vi "Automatic Teller Machine (ATM).vi"() -> ()   [LabVIEW 2020]
doc: "This VI simulates the behavior of an Automated Teller Machine (ATM)."
uses:
  Controls/Machine States.ctl
  Controls/Controls-Indicators References.ctl
  Controls/ATM Message Types.ctl
  Controls/Previous State.ctl
panel:
  in  "Enter":bool
  in  "User Input":string
  in  "Right Buttons":T1
  out "Right Menu":T2
  in  "Left Buttons":T1
  out "Left Menu":T2
  in  "Card Simulator":bool
  out "ATM Messages":string
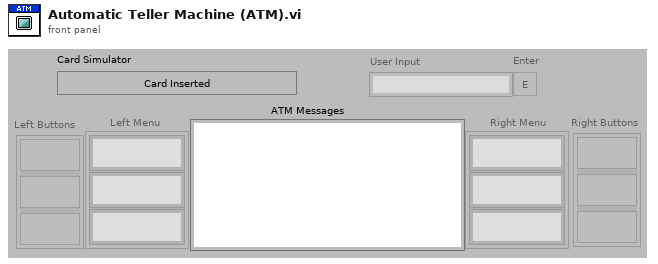
[diagram p1: front panel]
types:
  T1 = cluster{"Func Button":bool, "Func Button 2":bool, "Func Button 3":bool}
  T2 = cluster{"RFS String":string, "RFS String 2":string, "RFS String 3":string}
  T3 = typedef "Controls-Indicators References.ctl" = cluster{"Enter":refnum<vi>, "User Input":refnum<vi>, "Right Buttons":refnum<vi>, "Right Menu":refnum<vi>, "Left Buttons":refnum<vi>, "Left Menu":refnum<vi>, "Card Simulator":refnum<vi>, "ATM Messages":refnum<vi>}
  T4 = typedef "Machine States.ctl" = enum16{"Initialize", "Account Verification", "Deposit", "Withdraw", "None", "Fast Cash", "Balance Inquiry", "Wait User Action", "Return Card"}
  T5 = typedef "Previous State.ctl" = enum16{"Initialize", "Wait User Action", "Account Verification", "Wait Withdraw", "Wait Deposit"}
  T6 = typedef "ATM Message Types.ctl" = enum16{"Welcome", "Main Menu", "Account Verification Failed", "Session Terminate Message", "Deposit ", "Deposit Completed", "Withdrawal", "Withdrawal Complete", "Withdrawal Failed", "Balance Inquiry"}
  T7 = cluster{"Balance":dbl, "Name":string, "Password":string}
  T8 = enum8{"Enabled", "Disabled", "Disabled and Grayed Out"}
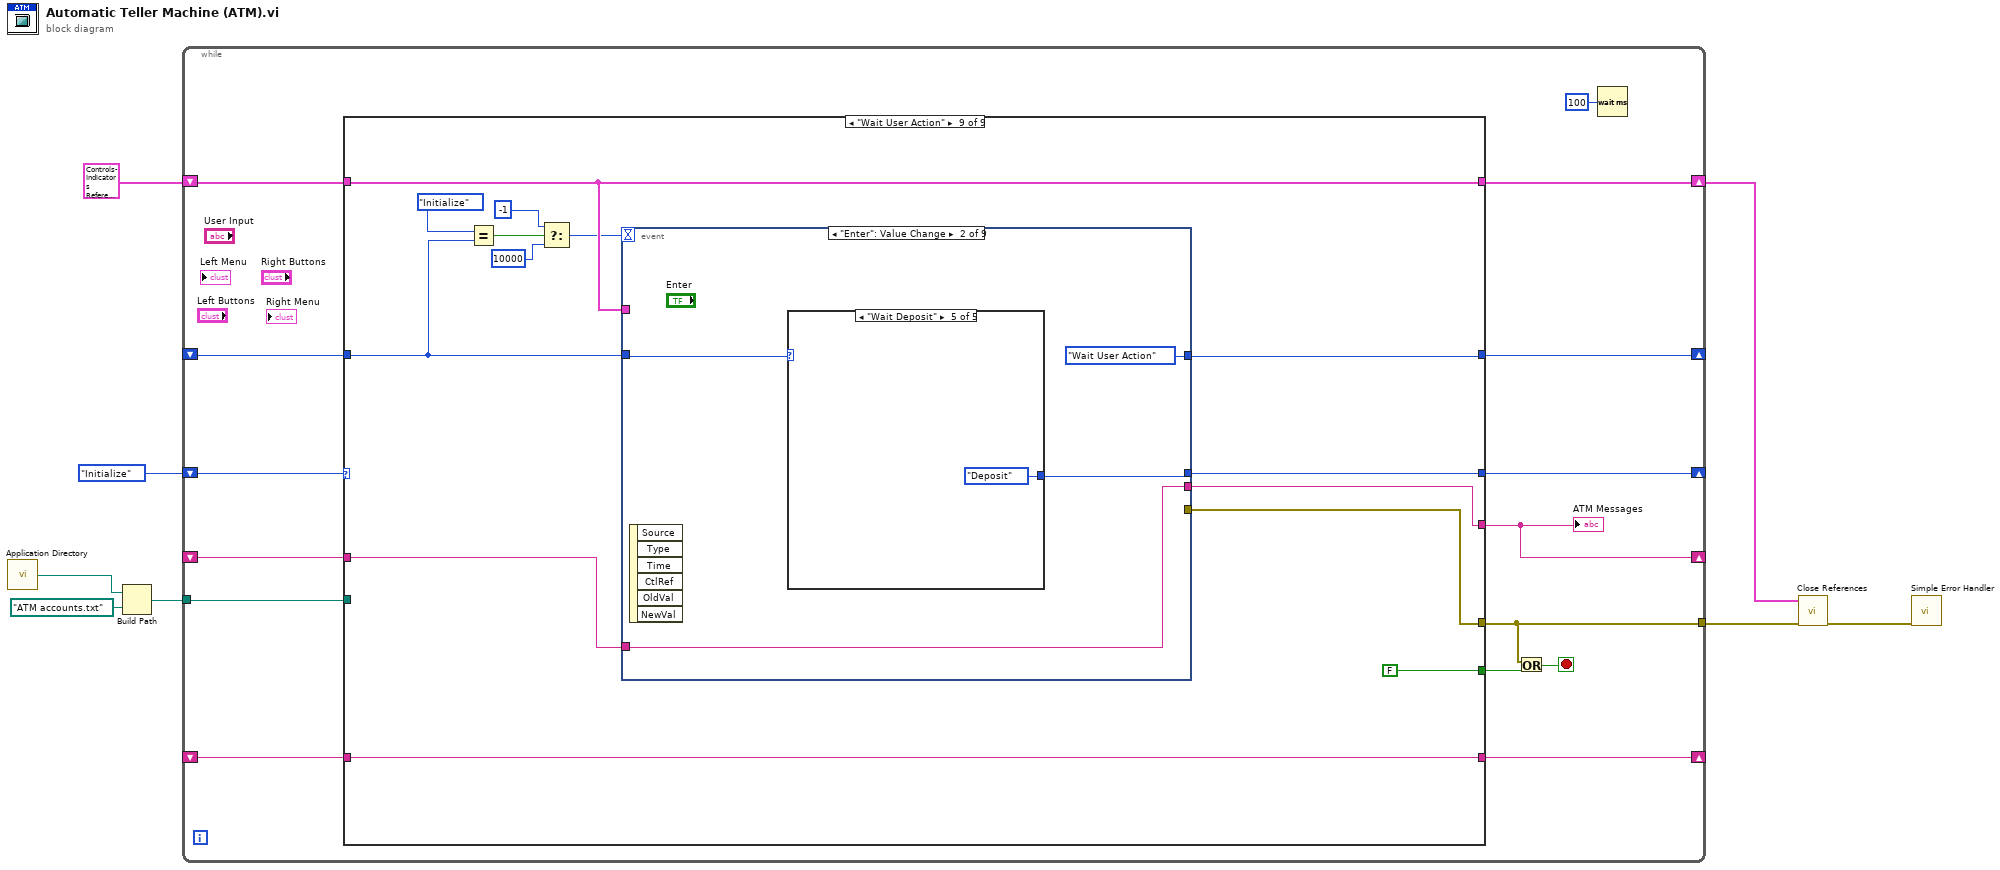
[diagram p0: block diagram]
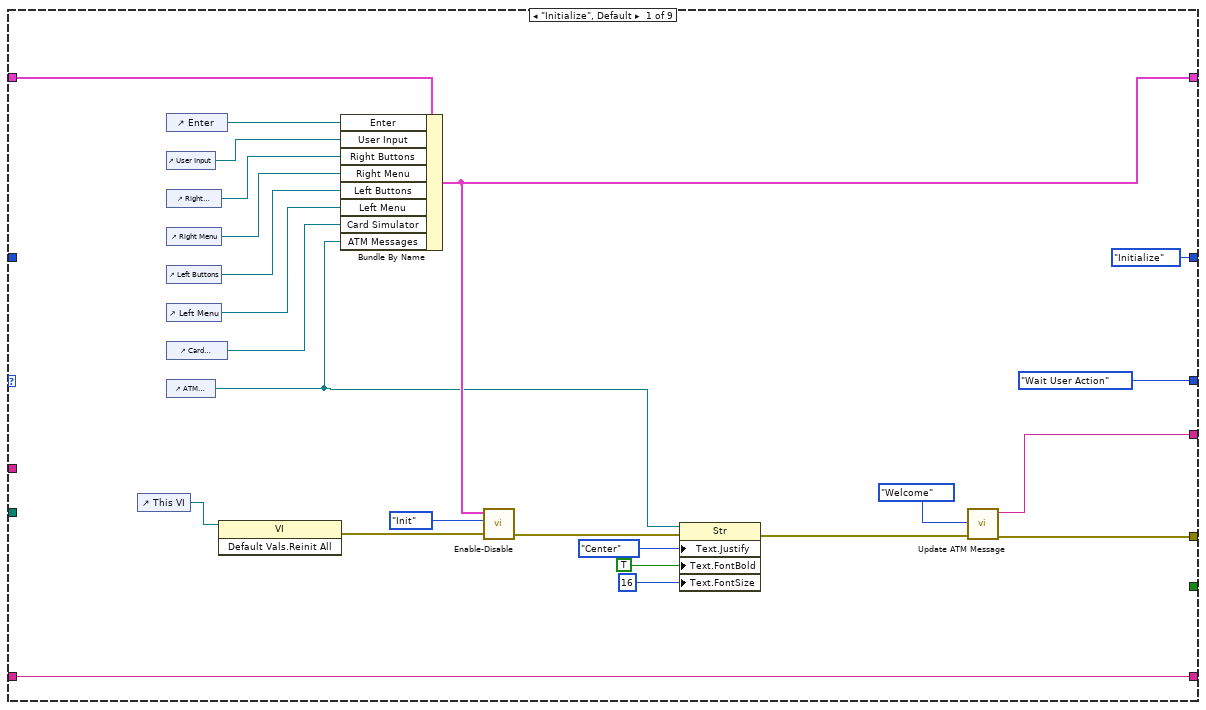
[diagram p2: hidden frame]
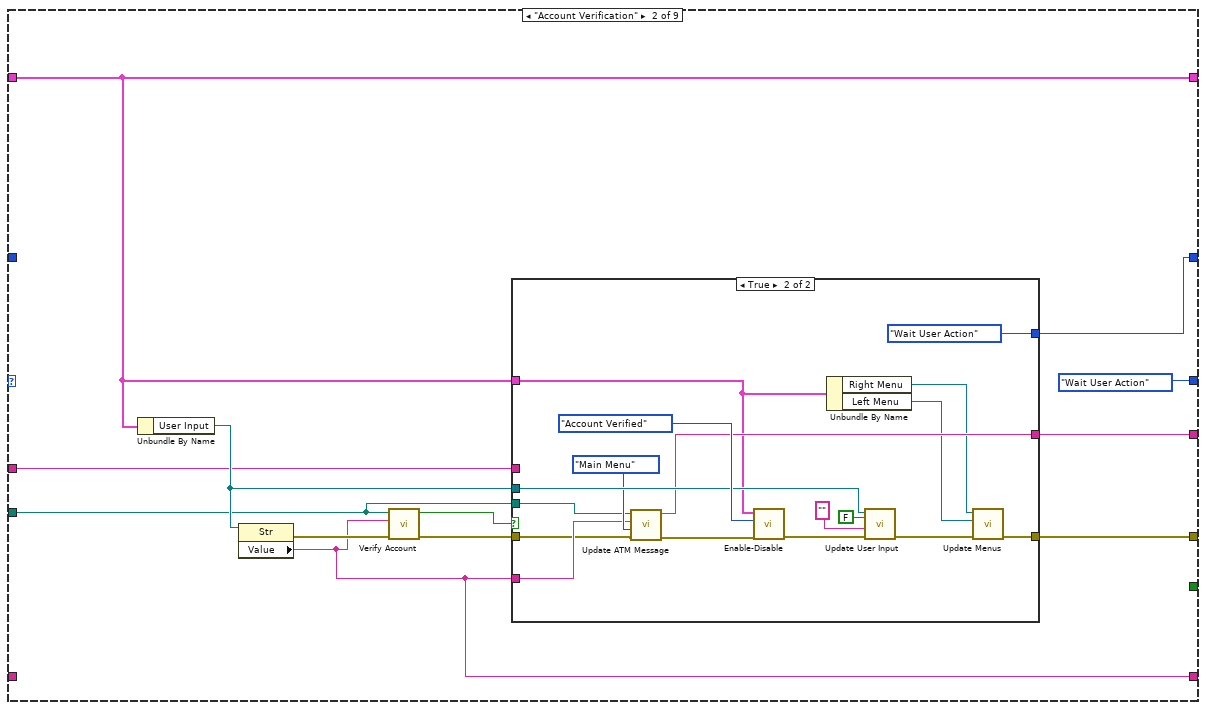
[diagram p3: hidden frame]
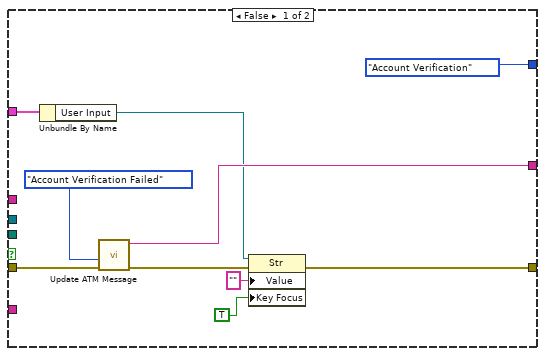
[diagram p4: hidden frame]
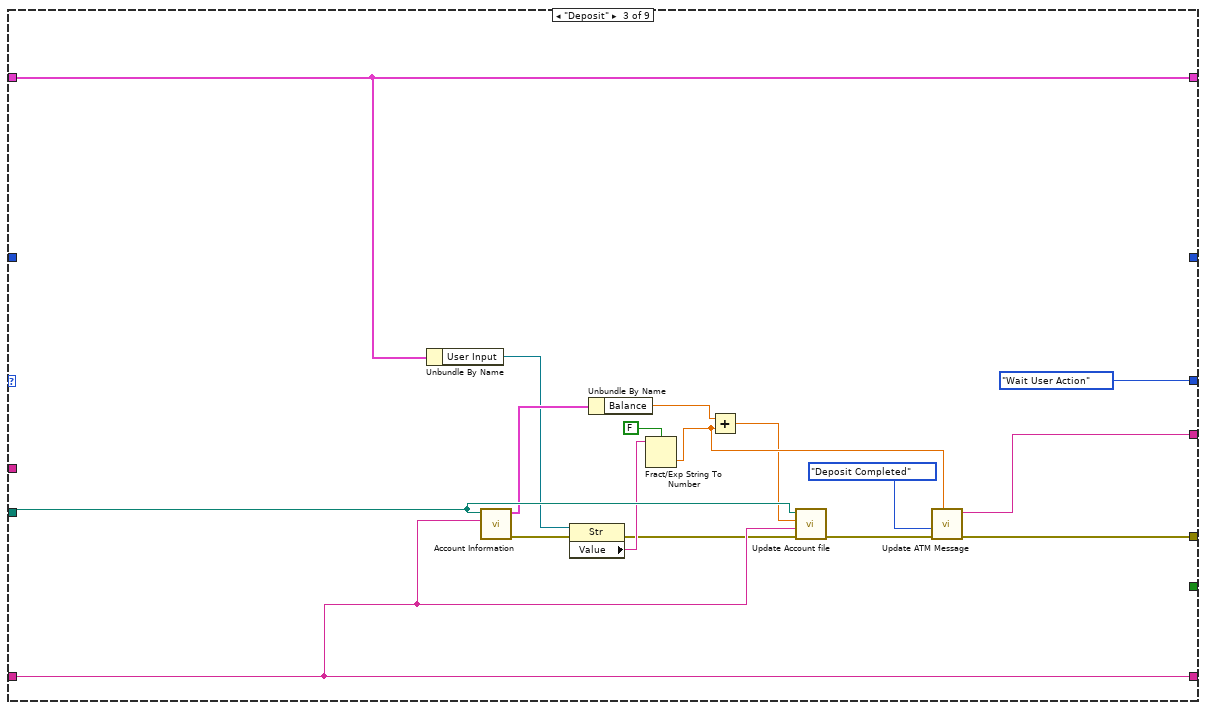
[diagram p5: hidden frame]
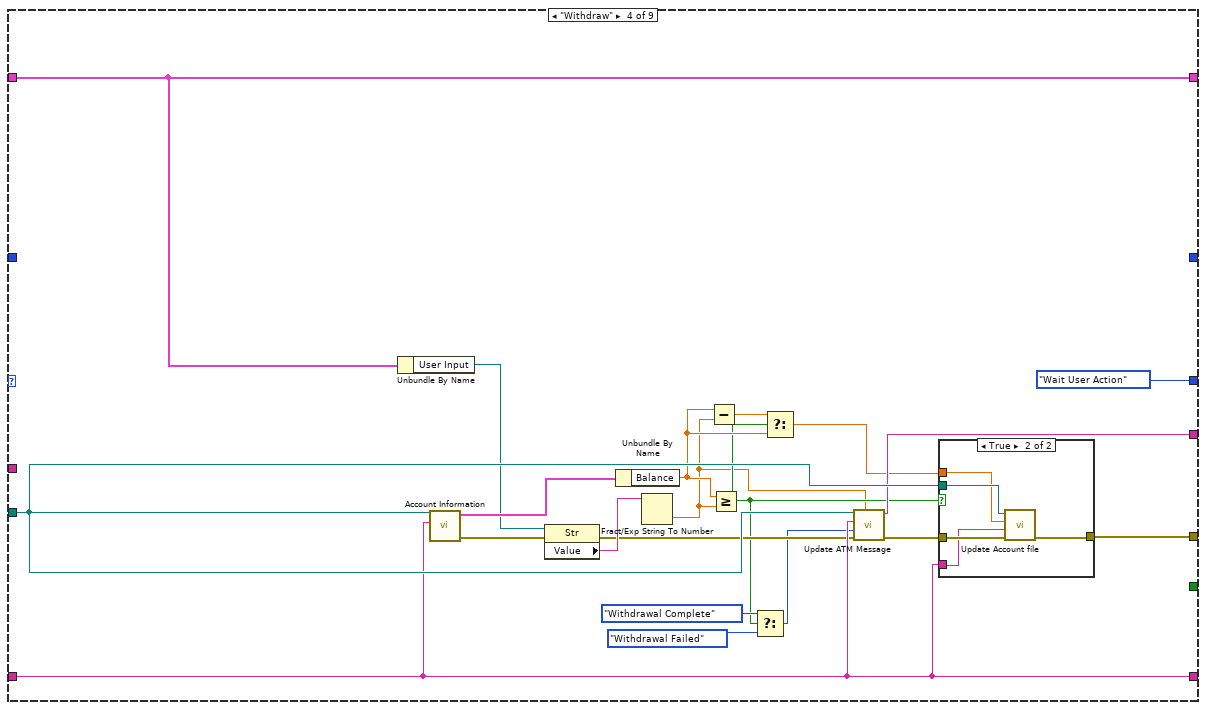
[diagram p6: hidden frame]
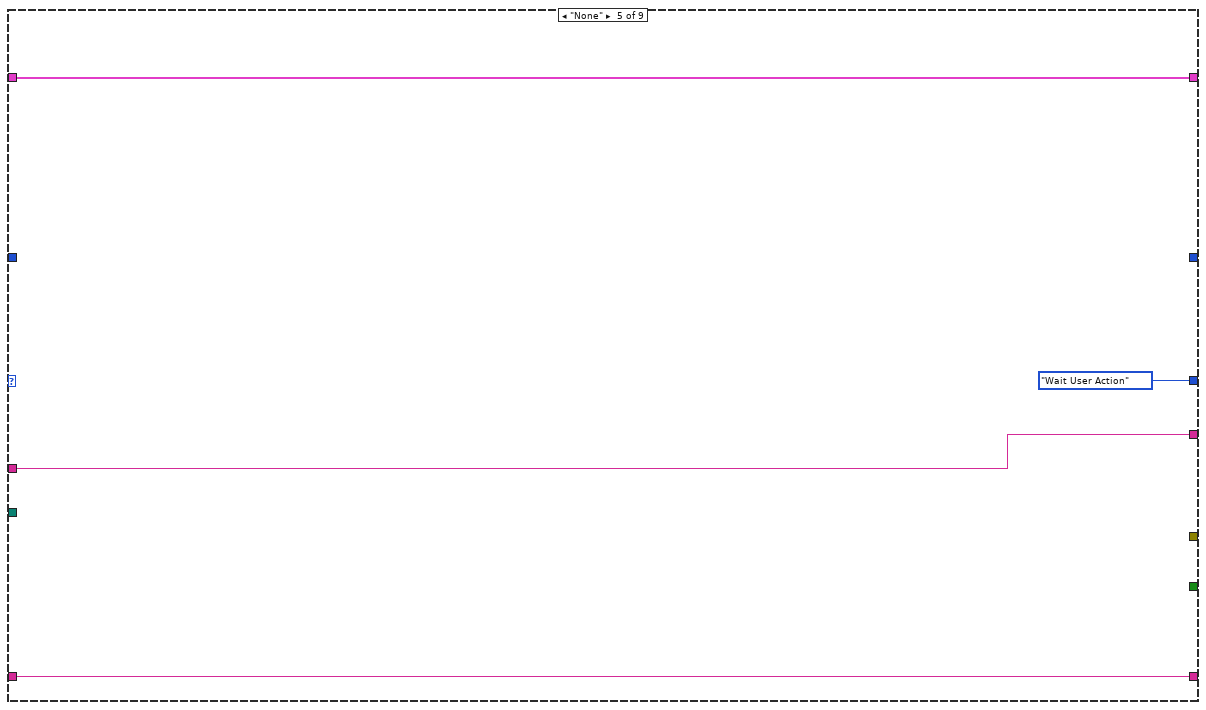
[diagram p8: hidden frame]
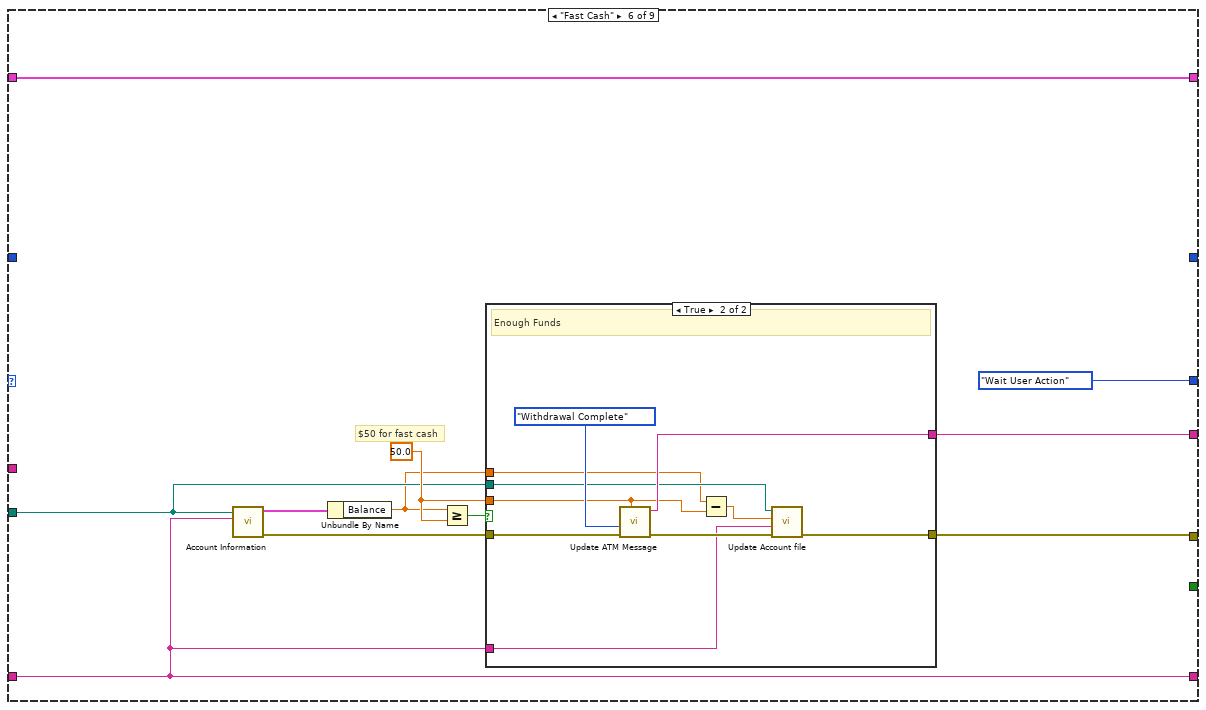
[diagram p9: hidden frame]
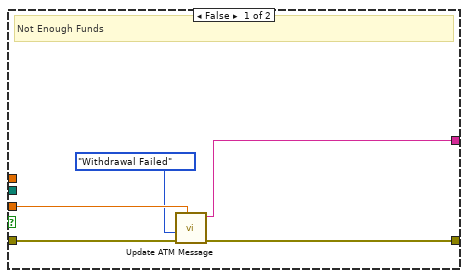
[diagram p10: hidden frame]
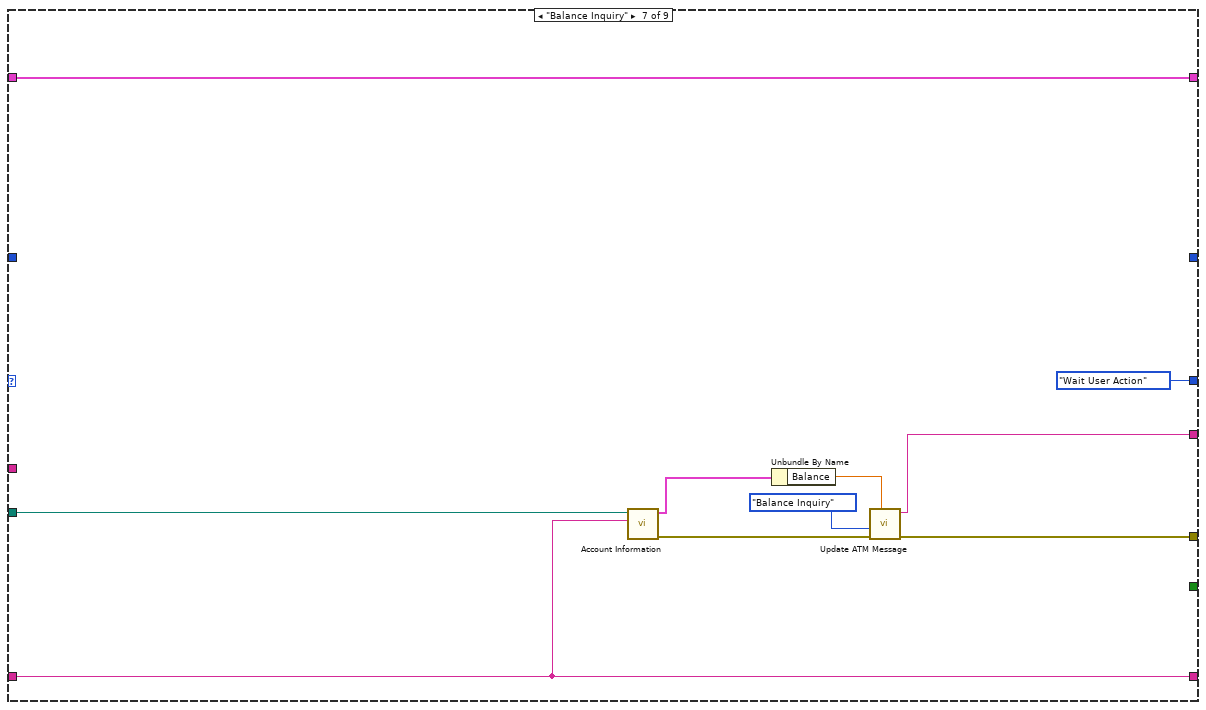
[diagram p11: hidden frame]
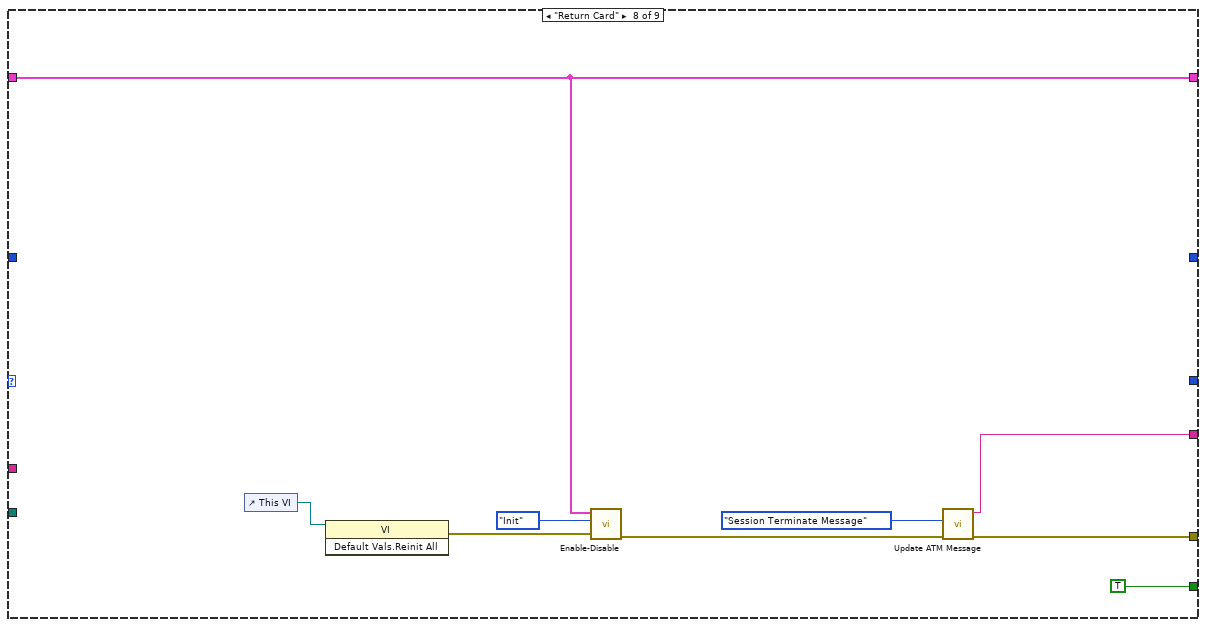
[diagram p12: hidden frame]
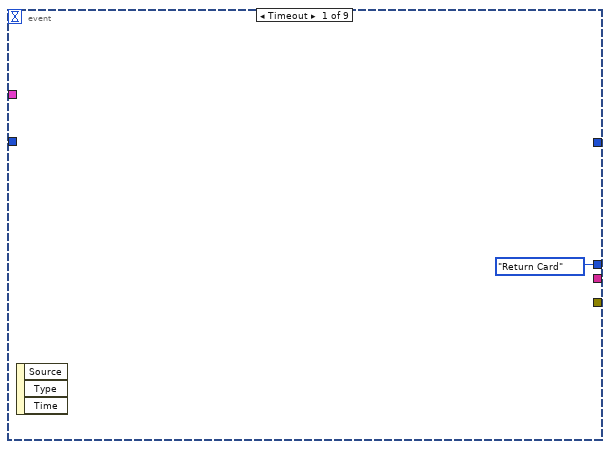
[diagram p13: hidden frame]
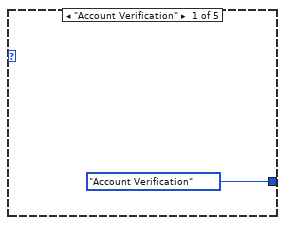
[diagram p14: hidden frame]
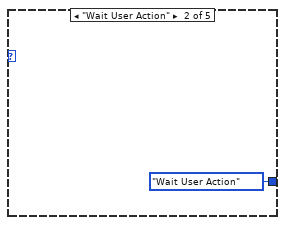
[diagram p15: hidden frame]
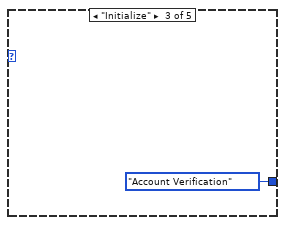
[diagram p16: hidden frame]
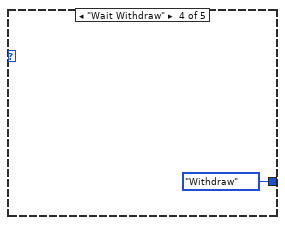
[diagram p17: hidden frame]
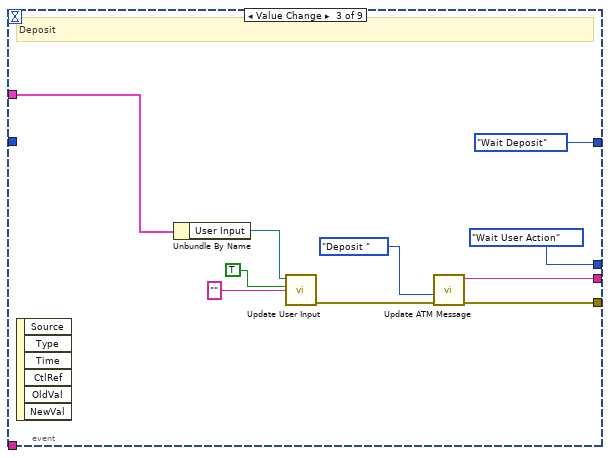
[diagram p18: hidden frame]
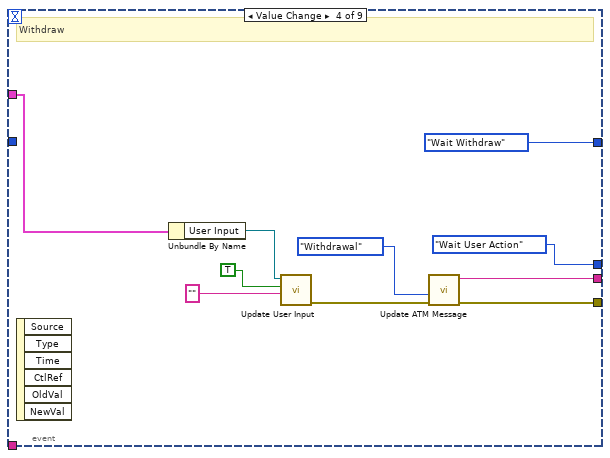
[diagram p19: hidden frame]
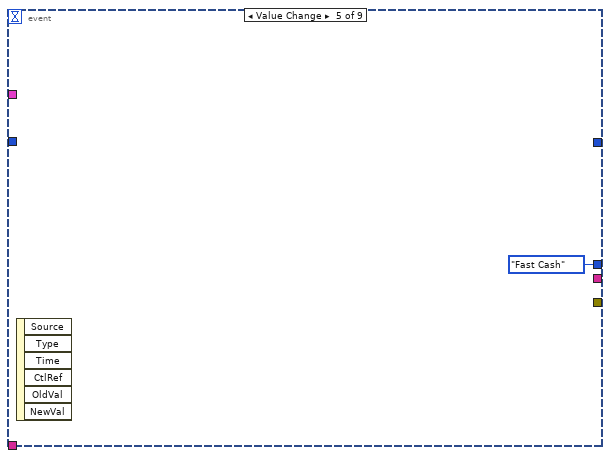
[diagram p20: hidden frame]
diagram:
  n1 = call <vilib>:"Application Directory.vi"() -> ("Application Directory"=w4:path)
  n2 = Build Path(base path=w4, name or relative path=path "ATM accounts.txt") -> (appended path=w5:path)
  n3 = while {
    shift-right: [w19] -> _
    shift-left: Machine_States."Initialize" ("Enum") -> [w23]
    shift-right: [w18] -> _
    shift-left: _ -> [w17]
    shift-right: [w20] -> w3
    shift-left: T3 {"Enter"=refnum, "User Input"=refnum, "Right Buttons"=refnum, "Right Menu"=refnum, "Left Buttons"=refnum, "Left Menu"=refnum, "Card Simulator"=refnum, "ATM Messages"=refnum} ("input cluster") -> [w21]
    tunnel: w5 -> [w16]
    shift-right: [w14] -> _
    shift-left: _ -> [w13]
    shift-right: [w10] -> _
    shift-left: _ -> [w11]
    tunnel: [w9] -> w2
    stop <- w22 stop-if-true
    n4 = case shown="\"Wait User Action\"" w23 {
      tunnel: [w45 w56 w102 w120 _ w135 w168 w177 w188] -> w9
      tunnel: w21 -> [w47 w51 w99 w121 w133 w144 w169 w170 w190]
      tunnel: [w44 w51 w99 w121 w133 w144 w169 w170 w190] -> w20
      tunnel: [w46 w53 w101 w119 w131 w139 w160 w176 w180] -> w18
      tunnel: [Machine_States."Wait User Action" ("Enum") Machine_States."Wait User Action" ("Enum") Machine_States."Wait User Action" ("Enum") Machine_States."Wait User Action" ("Enum") Machine_States."Wait User Action" ("Enum") Machine_States."Wait User Action" ("Enum") Machine_States."Wait User Action" ("Enum") _ w192] -> w19
      tunnel: w17 -> [_ w52 _ _ w131 _ _ _ w179]
      tunnel: w16 -> [_ w54 w103 w123 _ w138 w165 _ _]
      tunnel: [_ _ _ _ _ _ _ TRUE ("x .or. y?") FALSE ("x .or. y?")] -> w15
      tunnel: [w25 w50 w98 w122 w132 w137 w166 _ w189] -> w14
      tunnel: w13 -> [w25 _ w98 w122 w132 w137 w166 _ w189]
      tunnel: w11 -> [_ _ _ _ _ _ _ _ w187]
      tunnel: [Previous_State."Initialize" w49 _ _ _ _ _ _ w181] -> w10
      frame "Initialize", Default {
        n5 = control-ref of="This VI"() -> (w41:refnum<vi>)
        n6 = control-ref of="Enter"() -> (w32:refnum<vi>)
        n7 = control-ref of="User Input"() -> (w31:refnum<vi>)
        n8 = control-ref of="Right Buttons"() -> (w30:refnum<vi>)
        n9 = control-ref of="Right Menu"() -> (w29:refnum<vi>)
        n10 = control-ref of="Left Buttons"() -> (w28:refnum<vi>)
        n11 = control-ref of="Left Menu"() -> (w27:refnum<vi>)
        n12 = control-ref of="Card Simulator"() -> (w26:refnum<vi>)
        n13 = control-ref of="ATM Messages"() -> (w43:refnum<vi>)
        n14 = invoke class="VI" method="Default Vals.Reinit All"(reference=w41) -> (error out=w40:errorcluster)  [unwired: 2 in, 2 out]
        n15 = Bundle By Name(cluster=w47, "Enter"=w32, "User Input"=w31, "Right Buttons"=w30, "Right Menu"=w29, "Left Buttons"=w28, "Left Menu"=w27, "Card Simulator"=w26, "ATM Messages"=w43) -> (w44:T3)
        n16 = call "Enable-Disable.vi"("error in (no error)"=w40, "State"=enum16{"Init", "Account Verified"}."Init", "Control/Indicator References"=w44) -> ("error out"=w38:errorcluster)  [unwired: 8 in]
        n17 = property class="Str"(reference=w43, error in=w38, "Text.Justify"=enum16{"Left", "Center", "Right"}."Center" ("Text.Justification"), "Text.FontBold"=TRUE ("Text.Font:Bold"), "Text.FontSize"=u32 16 ("Text.Font:Size")) -> (error out=w33:errorcluster)  [unwired: 1 out]
        n18 = call "Update ATM Message.vi"("error in (no error)"=w33, "ATM Message Type"=ATM_Message_Types."Welcome") -> ("error out"=w45:errorcluster, "ATM Messages"=w46:string)  [unwired: 8 in]
      }
      frame "Account Verification" {
        n19 = Unbundle By Name(w51) -> ("User Input"=w55:refnum<vi>)
        n20 = property class="Str"(reference=w55) -> (error out=w59:errorcluster, "Value"=w50:string)  [unwired: 1 in, 1 out]
        n21 = call "Verify Account.vi"("error in (no error)"=w59, "Account"=w50, "Path Account File"=w54) -> ("error out"=w57:errorcluster, "Account exist?"=w58:bool)  [unwired: 7 in]
        n22 = case shown="True" w58 {
          tunnel: w57 -> [w66 w79]
          tunnel: [w61 w74] -> w56
          tunnel: w55 -> [_ w84]
          tunnel: w54 -> [_ w82]
          tunnel: w50 -> [_ w81]
          tunnel: [w67 w80] -> w53
          tunnel: w52 -> [_ _]
          tunnel: w51 -> [w69 w73]
          tunnel: [Previous_State."Account Verification" Previous_State."Wait User Action"] -> w49
          frame False {
            n23 = Unbundle By Name(w69) -> ("User Input"=w64:refnum<vi>)
            n24 = call "Update ATM Message.vi"("error in (no error)"=w66, "ATM Message Type"=ATM_Message_Types."Account Verification Failed") -> ("error out"=w65:errorcluster, "ATM Messages"=w67:string)  [unwired: 8 in]
            n25 = property class="Str"(reference=w64, error in=w65, "Value"="", "Key Focus"=TRUE) -> (error out=w61:errorcluster)  [unwired: 1 out]
          }
          frame True {
            n26 = call "Update ATM Message.vi"("error in (no error)"=w79, "ATM Message Type"=ATM_Message_Types."Main Menu", "Password"=w81, "Path Account File"=w82) -> ("error out"=w78:errorcluster, "ATM Messages"=w80:string)  [unwired: 6 in]
            n27 = call "Enable-Disable.vi"("error in (no error)"=w78, "State"=enum16{"Init", "Account Verified"}."Account Verified", "Control/Indicator References"=w73) -> ("error out"=w85:errorcluster)  [unwired: 8 in]
            n28 = Unbundle By Name(w73) -> ("Right Menu"=w72:refnum<vi>, "Left Menu"=w71:refnum<vi>)
            n29 = call "Update User Input.vi"("error in (no error)"=w85, "Value"="", "Key Focus"=FALSE, "User Input Reference"=w84) -> ("error out"=w75:errorcluster)  [unwired: 7 in]
            n30 = call "Update Menus.vi"("error in (no error)"=w75, "Left Menu"=w71, "Right Menu"=w72) -> ("error out"=w74:errorcluster)  [unwired: 8 in]
          }
        }
      }
      frame "Deposit" {
        n31 = Unbundle By Name(w99) -> ("User Input"=w96:refnum<vi>)
        n32 = call "Account Information.vi"("Password"=w98, "file path (dialog if empty)"=w103) -> ("error out"=w93:errorcluster, "Account Information"=w97:T7)  [unwired: 8 in]
        n33 = property class="Str"(reference=w96, error in=w93) -> (error out=w92:errorcluster, "Value"=w95:string)  [unwired: 1 out]
        n34 = Unbundle By Name(w97) -> ("Balance"=w91:dbl)
        n35 = Fract/Exp String To Number(use system decimal point (T)=FALSE, string=w95) -> (number=w88:dbl)  [unwired: 2 in, 1 out]
        n36 = Add(x=w91, y=w88) -> (x+y=w87:dbl)
        n37 = call "Update Account file.vi"("error in (no error)"=w92, "Account"=w98, "Balance"=w87, "name or relative path"=w103) -> ("error out"=w94:errorcluster)  [unwired: 7 in]
        n38 = call "Update ATM Message.vi"("Balance"=w88, "error in (no error)"=w94, "ATM Message Type"=ATM_Message_Types."Deposit Completed") -> ("error out"=w102:errorcluster, "ATM Messages"=w101:string)  [unwired: 7 in]
      }
      frame "Withdraw" {
        n39 = Unbundle By Name(w121) -> ("User Input"=w116:refnum<vi>)
        n40 = call "Account Information.vi"("Password"=w122, "file path (dialog if empty)"=w123) -> ("error out"=w117:errorcluster, "Account Information"=w118:T7)  [unwired: 8 in]
        n41 = property class="Str"(reference=w116, error in=w117) -> (error out=w114:errorcluster, "Value"=w115:string)  [unwired: 1 out]
        n42 = Unbundle By Name(w118) -> ("Balance"=w109:dbl)
        n43 = Fract/Exp String To Number(string=w115) -> (number=w104:dbl)  [unwired: 3 in, 1 out]
        n44 = Subtract(x=w109, y=w104) -> (x-y=w110:dbl)
        n45 = Greater Or Equal?(x=w109, y=w104) -> (x >= y?=w108:bool)
        n46 = Select(t=ATM_Message_Types."Withdrawal Complete" ("ATM Message Type"), s=w108, f=ATM_Message_Types."Withdrawal Failed" ("ATM Message Type")) -> (s? t:f=w111:T6)
        n47 = Select(t=w110, s=w108, f=w109) -> (s? t:f=w105:dbl)
        n48 = call "Update ATM Message.vi"("Balance"=w104, "error in (no error)"=w114, "ATM Message Type"=w111, "Password"=w122, "Path Account File"=w123) -> ("error out"=w107:errorcluster, "ATM Messages"=w119:string)  [unwired: 5 in]
        n49 = case shown="True" w108 {
          tunnel: w107 -> [w124 w129]
          tunnel: [w124 w128] -> w120
          tunnel: w123 -> [_ w127]
          tunnel: w105 -> [_ w126]
          tunnel: w122 -> [_ w125]
          frame False {
          }
          frame True {
            n50 = call "Update Account file.vi"("error in (no error)"=w129, "Account"=w125, "Balance"=w126, "name or relative path"=w127) -> ("error out"=w128:errorcluster)  [unwired: 7 in]
          }
        }
      }
      frame "None" {
      }
      frame "Fast Cash" {
        w140 = 50.0 ("y")
        # "$50 for fast cash"
        n51 = call "Account Information.vi"("Password"=w137, "file path (dialog if empty)"=w138) -> ("error out"=w142:errorcluster, "Account Information"=w143:T7)  [unwired: 8 in]
        n52 = Unbundle By Name(w143) -> ("Balance"=w136:dbl)
        n53 = Greater Or Equal?(x=w136, y=w140) -> (x >= y?=w141:bool)
        n54 = case shown="True" w141 {
          tunnel: w142 -> [w149 w158]
          tunnel: w140 -> [w148 w150]
          tunnel: [w146 w157] -> w139
          tunnel: [w145 w155] -> w135
          tunnel: w138 -> [_ w154]
          tunnel: w137 -> [_ w153]
          tunnel: w136 -> [_ w151]
          frame False {
            # "Not Enough Funds"
            n55 = call "Update ATM Message.vi"("Balance"=w148, "error in (no error)"=w149, "ATM Message Type"=ATM_Message_Types."Withdrawal Failed") -> ("error out"=w145:errorcluster, "ATM Messages"=w146:string)  [unwired: 7 in]
          }
          frame True {
            # "Enough Funds"
            n56 = call "Update ATM Message.vi"("Balance"=w150, "error in (no error)"=w158, "ATM Message Type"=ATM_Message_Types."Withdrawal Complete") -> ("error out"=w156:errorcluster, "ATM Messages"=w157:string)  [unwired: 7 in]
            n57 = Subtract(x=w151, y=w150) -> (x-y=w152:dbl)
            n58 = call "Update Account file.vi"("error in (no error)"=w156, "Account"=w153, "Balance"=w152, "name or relative path"=w154) -> ("error out"=w155:errorcluster)  [unwired: 7 in]
          }
        }
      }
      frame "Balance Inquiry" {
        n59 = call "Account Information.vi"("Password"=w166, "file path (dialog if empty)"=w165) -> ("error out"=w167:errorcluster, "Account Information"=w164:T7)  [unwired: 8 in]
        n60 = Unbundle By Name(w164) -> ("Balance"=w163:dbl)
        n61 = call "Update ATM Message.vi"("Balance"=w163, "error in (no error)"=w167, "ATM Message Type"=ATM_Message_Types."Balance Inquiry") -> ("error out"=w168:errorcluster, "ATM Messages"=w160:string)  [unwired: 7 in]
      }
      frame "Return Card" {
        n62 = control-ref of="This VI"() -> (w174:refnum<vi>)
        n63 = invoke class="VI" method="Default Vals.Reinit All"(reference=w174) -> (error out=w173:errorcluster)  [unwired: 2 in, 2 out]
        n64 = call "Enable-Disable.vi"("error in (no error)"=w173, "State"=enum16{"Init", "Account Verified"}."Init", "Control/Indicator References"=w170) -> ("error out"=w171:errorcluster)  [unwired: 8 in]
        n65 = call "Update ATM Message.vi"("error in (no error)"=w171, "ATM Message Type"=ATM_Message_Types."Session Terminate Message") -> ("error out"=w177:errorcluster, "ATM Messages"=w176:string)  [unwired: 8 in]
      }
      frame "Wait User Action" {
        n66 = Equal?(x=Previous_State."Initialize", y=w187) -> (x = y?=w185:bool)
        n67 = Select(t=-1, s=w185, f=10000) -> (s? t:f=w182:i32)
        n68 = event shown="[1] \"Enter\": Value Change" {
          selector: _ -> [_ _ _ _ _ _ _ _ _]
          dyn-events: _ -> [_ _ _ _ _ _ _ _ _]
          timeout: w182 -> [_ _ _ _ _ _ _ _ _]
          tunnel: w190 -> [_ _ w206 w214 _ _ _ _ w231]
          tunnel: [Machine_States."Return Card" ("Enum") w196 Machine_States."Wait User Action" ("Enum") Machine_States."Wait User Action" ("Enum") Machine_States."Fast Cash" ("Enum") Machine_States."None" ("Enum") Machine_States."Balance Inquiry" ("Enum") Machine_States."Return Card" ("Enum") Machine_States."Wait User Action" ("Enum")] -> w192
          tunnel: w187 -> [_ w197 _ _ _ _ _ _ _]
          tunnel: [_ _ w207 w218 _ _ _ _ w232] -> w188
          tunnel: [_ Previous_State."Wait User Action" Previous_State."Wait Deposit" Previous_State."Wait Withdraw" _ _ _ _ Previous_State."Account Verification"] -> w181
          tunnel: [_ w195 w205 w217 _ w224 _ _ w228] -> w180
          tunnel: w179 -> [_ w195 _ _ _ w224 _ _ w228]
          event Timeout {
            n69 = event-data() -> ()  [unwired: 1 in, 3 out]
          }
          event "Enter": Value Change {
            n70 = event-data() -> ()  [unwired: 1 in, 6 out]
            n71 = case shown="\"Wait Deposit\"" w197 {
              tunnel: [Machine_States."Account Verification" ("Enum") Machine_States."Wait User Action" ("Enum") Machine_States."Account Verification" ("Enum") Machine_States."Withdraw" ("Enum") Machine_States."Deposit" ("Enum")] -> w196
              frame "Account Verification" {
              }
              frame "Wait User Action" {
              }
              frame "Initialize" {
              }
              frame "Wait Withdraw" {
              }
              frame "Wait Deposit" {
              }
            }
          }
          event "Right Buttons.Func Button": Value Change {
            # "Deposit"
            n72 = event-data() -> ()  [unwired: 1 in, 6 out]
            n73 = Unbundle By Name(w206) -> ("User Input"=w210:refnum<vi>)
            n74 = call "Update User Input.vi"("Value"="", "Key Focus"=TRUE, "User Input Reference"=w210) -> ("error out"=w211:errorcluster)  [unwired: 8 in]
            n75 = call "Update ATM Message.vi"("error in (no error)"=w211, "ATM Message Type"=ATM_Message_Types."Deposit ") -> ("error out"=w207:errorcluster, "ATM Messages"=w205:string)  [unwired: 8 in]
          }
          event "Right Buttons.Func Button 2": Value Change {
            # "Withdraw"
            n76 = event-data() -> ()  [unwired: 1 in, 6 out]
            n77 = Unbundle By Name(w214) -> ("User Input"=w213:refnum<vi>)
            n78 = call "Update User Input.vi"("Value"="", "Key Focus"=TRUE, "User Input Reference"=w213) -> ("error out"=w221:errorcluster)  [unwired: 8 in]
            n79 = call "Update ATM Message.vi"("error in (no error)"=w221, "ATM Message Type"=ATM_Message_Types."Withdrawal") -> ("error out"=w218:errorcluster, "ATM Messages"=w217:string)  [unwired: 8 in]
          }
          event "Right Buttons.Func Button 3": Value Change {
            n80 = event-data() -> ()  [unwired: 1 in, 6 out]
          }
          event "Left Buttons.Func Button": Value Change {
            # "None"
            n81 = event-data() -> ()  [unwired: 1 in, 6 out]
          }
          event "Left Buttons.Func Button 2": Value Change {
            # "Balance Inquiry"
            n82 = event-data() -> ()  [unwired: 1 in, 6 out]
          }
          event "Left Buttons.Func Button 3": Value Change {
            # "Return Card & Terminate"
            n83 = event-data() -> ()  [unwired: 1 in, 6 out]
          }
          event "Card Simulator": Value Change {
            w240 = T8."Enabled" ("Disabled")
            n84 = event-data() -> ()  [unwired: 1 in, 6 out]
            n85 = Unbundle By Name(w231) -> ("User Input"=w235:refnum<vi>, "Enter"=w234:refnum<vi>, "Card Simulator"=w233:refnum<vi>)
            n86 = property class="Bool (strict)"(reference=w233, "BoolText.Text"="Card Inserted" ("Boolean Text.Text")) -> (error out=w237:errorcluster)  [unwired: 1 in, 1 out]
            n87 = property class="Bool"(reference=w234, "DisabledEnum"=w240) -> (error out=w238:errorcluster)  [unwired: 1 in, 1 out]
            n88 = property class="Str"(reference=w235, "DisabledEnum"=w240, "Key Focus"=TRUE) -> (error out=w239:errorcluster)  [unwired: 1 in, 1 out]
            n89 = Merge Errors(w239, w238, w237) -> (w232:errorcluster)
          }
        }
      }
    }
    "ATM Messages" <- w18
    n90 = Or(x=w9, y=w15) -> (x .or. y?=w22:bool)
    n91 = Wait (ms)(milliseconds to wait=u32 100) -> ()  [unwired: 1 out]
  }
  n92 = call "Close References.vi"("error in"=w2, "input cluster"=w3) -> ("error out"=w1:errorcluster)  [unwired: 9 in]
  n93 = call <vilib>:"Simple Error Handler.vi"("error in (no error)"=w1) -> ()  [unwired: 4 in, 5 out]
